vi "Channel Mng Update Test Cases.vi"() -> (0 "error out":errorcluster, 2 "status":string, 3 "pass":bool)   [LabVIEW 2021]
uses:
  CIF_NIChn/Double/CIF_NIChn_Double.lvclass
  D:/dev/Packages/Channel_Manager/src/CIFChannels/CIFChannels.lvclass
  CIFChannels/Typedef/Direction.ctl
  CIFChannelMng.lvclass
  CIFChannels/CIFChannels.lvclass/CIFChannels.ctl
  CIFChannelMng.lvclass/CIFChannelMng.ctl
  ChannelCommon/Utilities/Add Error.vi
  CIFChannels/Accessors/Read Name.vi
  CIFChannels/Accessors/Read Custom Config Data.vi
  CIFChannels/Accessors/Read Type.vi
  CIFChannels/Accessors/Read Direction.vi
  Utilities/Get Channel Index by Name.vi
  CIFChannels/Accessors/Read Channel State.vi
  Utilities/Remove Channel by Index.vi
  CIFChannels/Accessors/Read Tag Forced.vi
  <vilib>/CIF Foundation/CIF Utilities/Errors/Append Error Location.vi
  CIFChannels/Accessors/Write Channel State.vi
  CIFChannels/Core/Set Force.vi
  CIFChannels/CIFChannels.lvclass
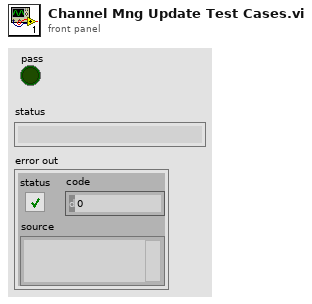
[diagram p1: front panel]
types:
  T1 = typedef "CIFChannels.lvclass/Direction.ctl" = enum16{"Publisher", "Subscriber"}
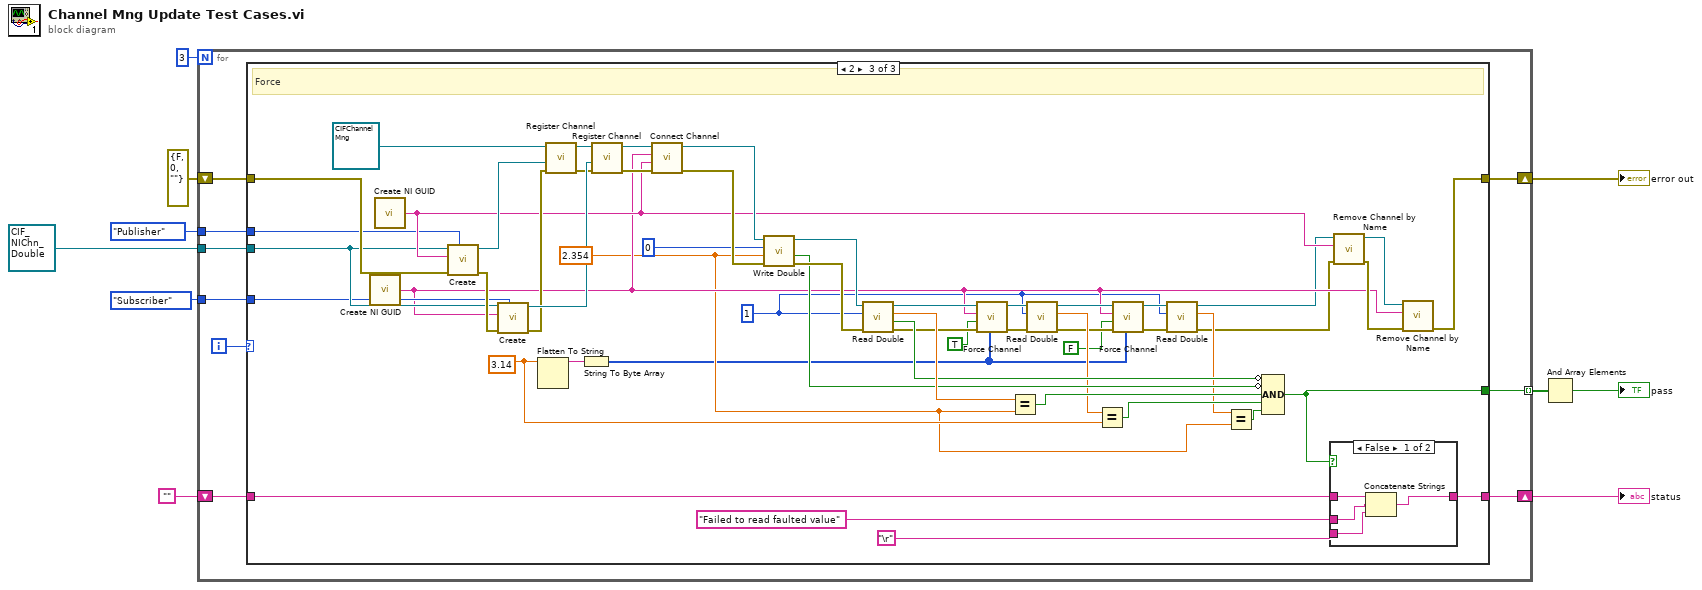
[diagram p0: block diagram]
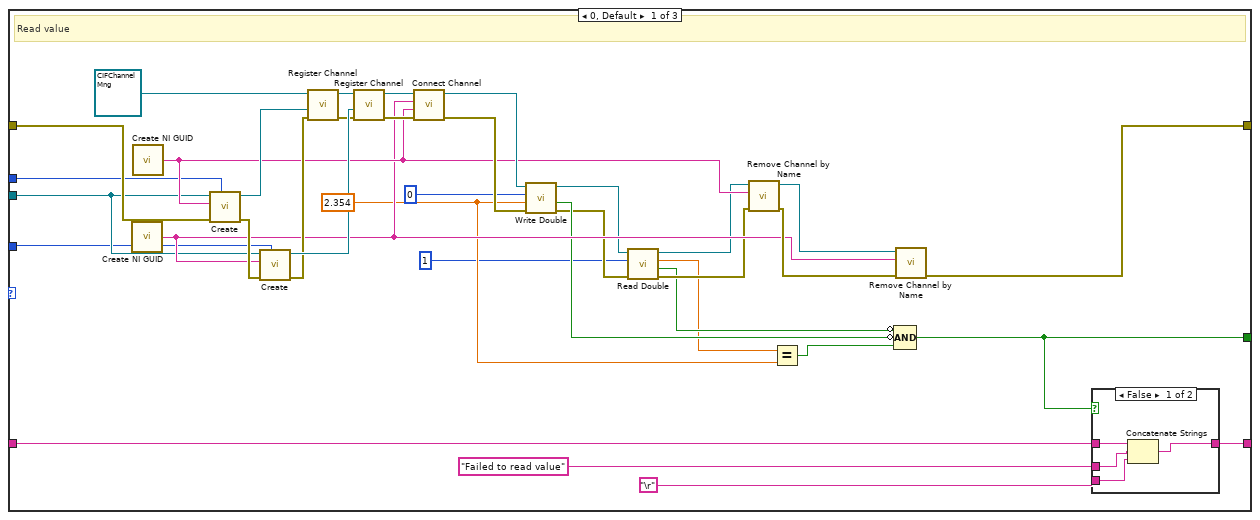
[diagram p2: hidden frame]
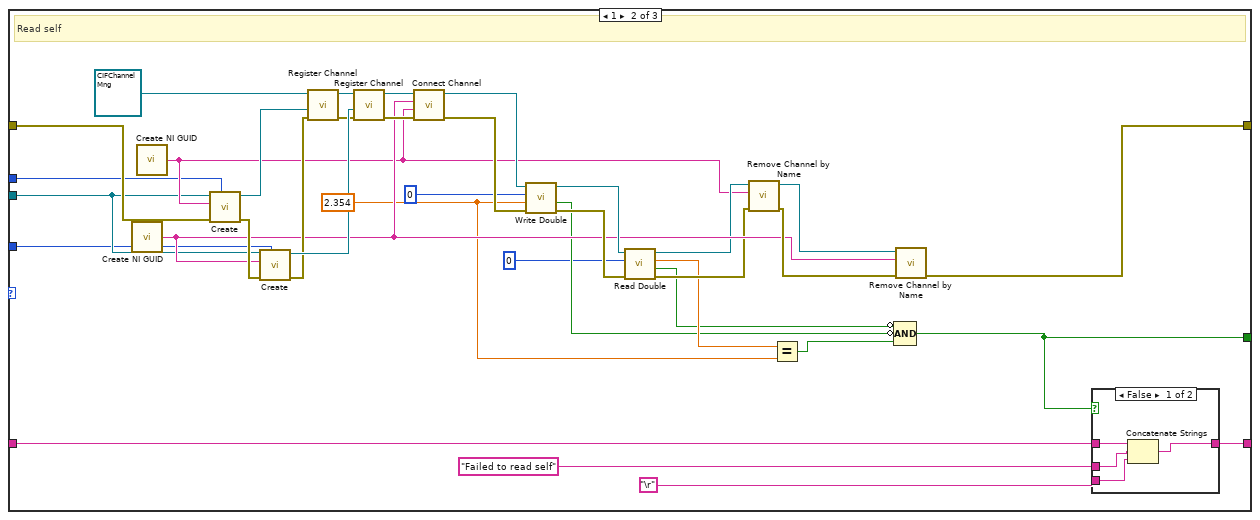
[diagram p4: hidden frame]
diagram:
  n1 = for {
    N: 3 -> [_]
    tunnel: [w19] -> w10 mode=indexing
    shift-right: [w17] -> w5
    shift-left: errorcluster {"status"=FALSE, "code"=0, "source"=""} ("error out") -> [w18]
    shift-right: [w14] -> w6
    shift-left: "" -> [w15]
    tunnel: refnum<class "CIF_NIChn_Double.lvclass"> refnum ("CIF_NIChn_Double.lvclass") -> [w13]
    tunnel: Direction."Subscriber" ("Direction") -> [w12]
    tunnel: Direction."Publisher" ("Direction") -> [w11]
    i -> [w16]
    n2 = case shown="2" w16 {
      tunnel: [w50 w91 w149] -> w19
      tunnel: w18 -> [w40 w81 w139]
      tunnel: [w34 w74 w132] -> w17
      tunnel: w15 -> [w55 w96 w154]
      tunnel: [w54 w95 w153] -> w14
      tunnel: w13 -> [w30 w65 w127]
      tunnel: w12 -> [w29 w64 w126]
      tunnel: w11 -> [w28 w63 w125]
      frame 0, Default {
        w32 = 2.354
        # "Read value"
        n3 = call <vilib>:"Create NI GUID.vi"() -> ("NI GUID"=w33:string)
        n4 = call <vilib>:"Create NI GUID.vi"() -> ("NI GUID"=w37:string)
        n5 = call-dynamic "Create.vi"("Direction"=w28, "error in (no error)"=w40, "Name"=w37, "CIFTag in"=w30) -> ("error out"=w45:errorcluster, "CIFTag out"=w44:refnum<class "CIF_NIChn_Double.lvclass">)  [unwired: 6 in]
        n6 = call-dynamic "Create.vi"("Direction"=w29, "error in (no error)"=w45, "Name"=w33, "CIFTag in"=w30) -> ("error out"=w46:errorcluster, "CIFTag out"=w49:refnum<class "CIF_NIChn_Double.lvclass">)  [unwired: 6 in]
        n7 = call "Register Channel.vi"("error in (no error)"=w46, "Channel"=w44, "CIFChannelMng in"=refnum<class "CIFChannelMng.lvclass"> refnum) -> ("error out"=w43:errorcluster, "CIFChannelMng out"=w42:refnum<class "CIFChannelMng.lvclass">)  [unwired: 7 in]
        n8 = call "Register Channel.vi"("error in (no error)"=w43, "Channel"=w49, "CIFChannelMng in"=w42) -> ("error out"=w48:errorcluster, "CIFChannelMng out"=w47:refnum<class "CIFChannelMng.lvclass">)  [unwired: 7 in]
        n9 = call "Connect Channel.vi"("error in (no error)"=w48, "Publisher Name"=w37, "Subscriber Name"=w33, "CIFChannelMng in"=w47) -> ("error out"=w38:errorcluster, "CIFChannelMng out"=w39:refnum<class "CIFChannelMng.lvclass">)  [unwired: 6 in]
        n10 = call "Write Double.vi"("error in (no error)"=w38, "Data"=w32, "Channel Index"=0, "CIFChannelMng in"=w39) -> ("error out"=w24:errorcluster, "timed out?"=w31:bool, "CIFChannelMng out"=w27:refnum<class "CIFChannelMng.lvclass">)  [unwired: 5 in]
        n11 = call "Read Double.vi"("error in (no error)"=w24, "Channel Index"=1 ("Index"), "CIFChannelMng in"=w27) -> ("error out"=w25:errorcluster, "timed out?"=w22:bool, "Data"=w21:dbl, "CIFChannelMng out"=w26:refnum<class "CIFChannelMng.lvclass">)  [unwired: 5 in]
        n12 = call "Remove Channel by Name.vi"("error in (no error)"=w25, "Channel Name"=w37, "CIFChannelMng in"=w26) -> ("error out"=w36:errorcluster, "CIFChannelMng out"=w35:refnum<class "CIFChannelMng.lvclass">)  [unwired: 7 in]
        n13 = Equal?(x=w21, y=w32) -> (x = y?=w51:bool)
        n14 = Compound Arithmetic op=AND(invert w22, invert w31, w51) -> (w50:bool)
        n15 = call "Remove Channel by Name.vi"("error in (no error)"=w36, "Channel Name"=w33, "CIFChannelMng in"=w35) -> ("error out"=w34:errorcluster)  [unwired: 7 in, 1 out]
        n16 = case shown="False" w50 {
          tunnel: w55 -> [w59 w60]
          tunnel: [w56 w60] -> w54
          tunnel: "Failed to read value" -> [w58 _]
          tunnel: "\r" -> [w57 _]
          frame False {
            n17 = Concatenate Strings(w59, w58, w57) -> (w56:string)
          }
          frame True {
          }
        }
      }
      frame 1 {
        w69 = 2.354
        # "Read self"
        n18 = call <vilib>:"Create NI GUID.vi"() -> ("NI GUID"=w73:string)
        n19 = call <vilib>:"Create NI GUID.vi"() -> ("NI GUID"=w66:string)
        n20 = call-dynamic "Create.vi"("Direction"=w63, "error in (no error)"=w81, "Name"=w66, "CIFTag in"=w65) -> ("error out"=w86:errorcluster, "CIFTag out"=w85:refnum<class "CIF_NIChn_Double.lvclass">)  [unwired: 6 in]
        n21 = call-dynamic "Create.vi"("Direction"=w64, "error in (no error)"=w86, "Name"=w73, "CIFTag in"=w65) -> ("error out"=w87:errorcluster, "CIFTag out"=w90:refnum<class "CIF_NIChn_Double.lvclass">)  [unwired: 6 in]
        n22 = call "Register Channel.vi"("error in (no error)"=w87, "Channel"=w85, "CIFChannelMng in"=refnum<class "CIFChannelMng.lvclass"> refnum) -> ("error out"=w84:errorcluster, "CIFChannelMng out"=w83:refnum<class "CIFChannelMng.lvclass">)  [unwired: 7 in]
        n23 = call "Register Channel.vi"("error in (no error)"=w84, "Channel"=w90, "CIFChannelMng in"=w83) -> ("error out"=w89:errorcluster, "CIFChannelMng out"=w88:refnum<class "CIFChannelMng.lvclass">)  [unwired: 7 in]
        n24 = call "Connect Channel.vi"("error in (no error)"=w89, "Publisher Name"=w66, "Subscriber Name"=w73, "CIFChannelMng in"=w88) -> ("error out"=w79:errorcluster, "CIFChannelMng out"=w80:refnum<class "CIFChannelMng.lvclass">)  [unwired: 6 in]
        n25 = call "Write Double.vi"("error in (no error)"=w79, "Data"=w69, "Channel Index"=0, "CIFChannelMng in"=w80) -> ("error out"=w78:errorcluster, "timed out?"=w67:bool, "CIFChannelMng out"=w77:refnum<class "CIFChannelMng.lvclass">)  [unwired: 5 in]
        n26 = call "Read Double.vi"("error in (no error)"=w78, "Channel Index"=0, "CIFChannelMng in"=w77) -> ("error out"=w72:errorcluster, "timed out?"=w68:bool, "Data"=w70:dbl, "CIFChannelMng out"=w71:refnum<class "CIFChannelMng.lvclass">)  [unwired: 5 in]
        n27 = call "Remove Channel by Name.vi"("error in (no error)"=w72, "Channel Name"=w66, "CIFChannelMng in"=w71) -> ("error out"=w76:errorcluster, "CIFChannelMng out"=w75:refnum<class "CIFChannelMng.lvclass">)  [unwired: 7 in]
        n28 = Equal?(x=w70, y=w69) -> (x = y?=w92:bool)
        n29 = Compound Arithmetic op=AND(invert w68, invert w67, w92) -> (w91:bool)
        n30 = call "Remove Channel by Name.vi"("error in (no error)"=w76, "Channel Name"=w73, "CIFChannelMng in"=w75) -> ("error out"=w74:errorcluster)  [unwired: 7 in, 1 out]
        n31 = case shown="False" w91 {
          tunnel: w96 -> [w100 w101]
          tunnel: [w97 w101] -> w95
          tunnel: "Failed to read self" -> [w99 _]
          tunnel: "\r" -> [w98 _]
          frame False {
            n32 = Concatenate Strings(w100, w99, w98) -> (w97:string)
          }
          frame True {
          }
        }
      }
      frame 2 {
        w115 = 3.14
        w108 = 1 ("Channel Index")
        w105 = 2.354
        # "Force"
        n33 = call <vilib>:"Create NI GUID.vi"() -> ("NI GUID"=w110:string)
        n34 = call <vilib>:"Create NI GUID.vi"() -> ("NI GUID"=w128:string)
        n35 = call-dynamic "Create.vi"("Direction"=w125, "error in (no error)"=w139, "Name"=w128, "CIFTag in"=w127) -> ("error out"=w144:errorcluster, "CIFTag out"=w143:refnum<class "CIF_NIChn_Double.lvclass">)  [unwired: 6 in]
        n36 = call-dynamic "Create.vi"("Direction"=w126, "error in (no error)"=w144, "Name"=w110, "CIFTag in"=w127) -> ("error out"=w145:errorcluster, "CIFTag out"=w148:refnum<class "CIF_NIChn_Double.lvclass">)  [unwired: 6 in]
        n37 = Flatten To String(anything=w115) -> (data string=w120:string)  [unwired: 3 in, 2 out]
        n38 = call "Register Channel.vi"("error in (no error)"=w145, "Channel"=w143, "CIFChannelMng in"=refnum<class "CIFChannelMng.lvclass"> refnum) -> ("error out"=w142:errorcluster, "CIFChannelMng out"=w141:refnum<class "CIFChannelMng.lvclass">)  [unwired: 7 in]
        n39 = String To Byte Array(string=w120) -> (unsigned byte array=w102:u8[])
        n40 = call "Register Channel.vi"("error in (no error)"=w142, "Channel"=w148, "CIFChannelMng in"=w141) -> ("error out"=w147:errorcluster, "CIFChannelMng out"=w146:refnum<class "CIFChannelMng.lvclass">)  [unwired: 7 in]
        n41 = call "Connect Channel.vi"("error in (no error)"=w147, "Publisher Name"=w128, "Subscriber Name"=w110, "CIFChannelMng in"=w146) -> ("error out"=w137:errorcluster, "CIFChannelMng out"=w138:refnum<class "CIFChannelMng.lvclass">)  [unwired: 6 in]
        n42 = call "Write Double.vi"("error in (no error)"=w137, "Data"=w105, "Channel Index"=0, "CIFChannelMng in"=w138) -> ("error out"=w136:errorcluster, "timed out?"=w129:bool, "CIFChannelMng out"=w135:refnum<class "CIFChannelMng.lvclass">)  [unwired: 5 in]
        n43 = call "Read Double.vi"("error in (no error)"=w136, "Channel Index"=w108, "CIFChannelMng in"=w135) -> ("error out"=w122:errorcluster, "timed out?"=w130:bool, "Data"=w131:dbl, "CIFChannelMng out"=w123:refnum<class "CIFChannelMng.lvclass">)  [unwired: 5 in]
        n44 = call "Force Channel.vi"("Force Data"=w102, "error in (no error)"=w122, "Force Active"=TRUE ("Fault Active"), "Subscriber Name"=w110, "CIFChannelMng in"=w123) -> ("error out"=w118:errorcluster, "CIFChannelMng out"=w119:refnum<class "CIFChannelMng.lvclass">)  [unwired: 5 in]
        n45 = Equal?(x=w131, y=w105) -> (x = y?=w150:bool)
        n46 = call "Read Double.vi"("error in (no error)"=w118, "Channel Index"=w108, "CIFChannelMng in"=w119) -> ("error out"=w113:errorcluster, "Data"=w116:dbl, "CIFChannelMng out"=w114:refnum<class "CIFChannelMng.lvclass">)  [unwired: 5 in, 1 out]
        n47 = Equal?(x=w116, y=w115) -> (x = y?=w117:bool)
        n48 = call "Force Channel.vi"("Force Data"=w102, "error in (no error)"=w113, "Force Active"=FALSE ("Fault Active"), "Subscriber Name"=w110, "CIFChannelMng in"=w114) -> ("error out"=w111:errorcluster, "CIFChannelMng out"=w112:refnum<class "CIFChannelMng.lvclass">)  [unwired: 5 in]
        n49 = call "Read Double.vi"("error in (no error)"=w111, "Channel Index"=w108, "CIFChannelMng in"=w112) -> ("error out"=w103:errorcluster, "Data"=w106:dbl, "CIFChannelMng out"=w104:refnum<class "CIFChannelMng.lvclass">)  [unwired: 5 in, 1 out]
        n50 = Equal?(x=w106, y=w105) -> (x = y?=w107:bool)
        n51 = Compound Arithmetic op=AND(invert w130, invert w129, w150, w117, w107) -> (w149:bool)
        n52 = case shown="False" w149 {
          tunnel: w154 -> [w158 w159]
          tunnel: [w155 w159] -> w153
          tunnel: "Failed to read faulted value" -> [w157 _]
          tunnel: "\r" -> [w156 _]
          frame False {
            n53 = Concatenate Strings(w158, w157, w156) -> (w155:string)
          }
          frame True {
          }
        }
        n54 = call "Remove Channel by Name.vi"("error in (no error)"=w103, "Channel Name"=w128, "CIFChannelMng in"=w104) -> ("error out"=w134:errorcluster, "CIFChannelMng out"=w133:refnum<class "CIFChannelMng.lvclass">)  [unwired: 7 in]
        n55 = call "Remove Channel by Name.vi"("error in (no error)"=w134, "Channel Name"=w110, "CIFChannelMng in"=w133) -> ("error out"=w132:errorcluster)  [unwired: 7 in, 1 out]
      }
    }
  }
  "error out" <- w5
  "status" <- w6
  n56 = And Array Elements(Boolean array=w10) -> (logical AND=→"pass":bool)
